vi "二级-位移-转换-滤波1.vi"(11 "Waveform":dbl) -> (3 "Filtered x":dbl)   [LabVIEW 2020]
uses:
  <vilib>/ptbypt/NI_PtbyPt.lvlib
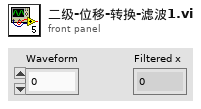
[diagram p1: front panel]
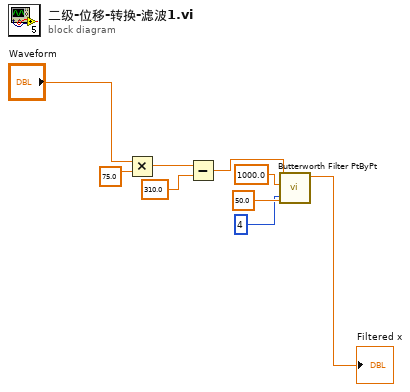
[diagram p0: block diagram]
diagram:
  n1 = Multiply(x="Waveform", y=75.0) -> (x*y=w7:dbl)
  n2 = Subtract(x=w7, y=310.0) -> (x-y=w5:dbl)
  n3 = call <vilib>:"Butterworth Filter PtByPt.vi"("order"=4, "low cutoff freq: fl"=50.0, "sampling freq: fs"=1000.0, "x"=w5) -> ("Filtered x"=→"Filtered x":dbl)  [unwired: 5 in, 1 out]
